vi "数据发送组合-20200825 (子VI).vi"(10 "枚举":T2(ring), 11 "插值后的数组元素":T1) -> (3 "字符串":string)   [LabVIEW 2016, in "数据传输系统-06.lvlib"]
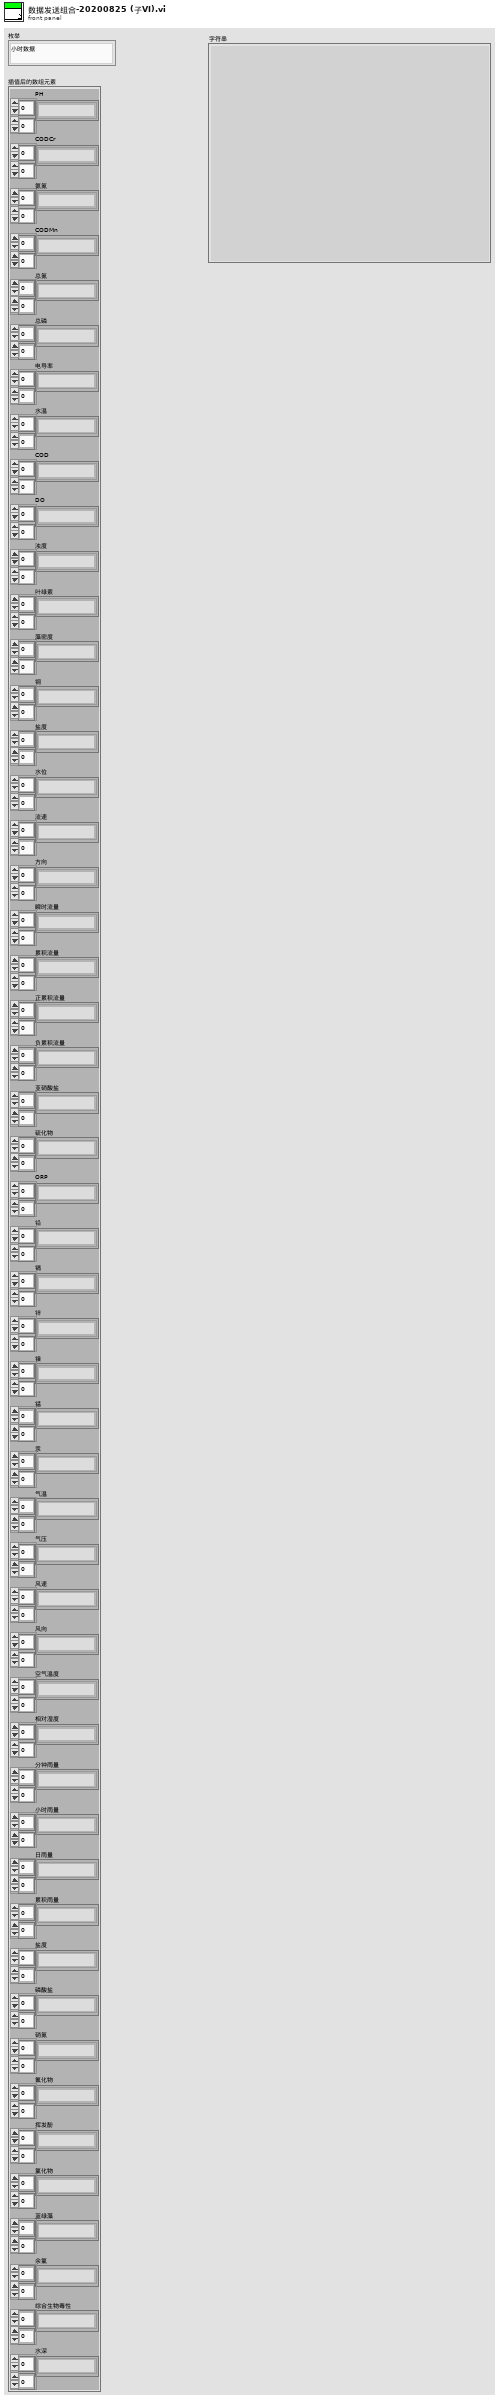
[diagram p1: front panel]
types:
  T1 = cluster{"PH":string[][], "CODCr":string[][], "氨氮":string[][], "CODMn":string[][], "总氮":string[][], "总磷":string[][], "电导率":string[][], "水温":string[][], "COD":string[][], "DO":string[][], "浊度":string[][], "叶绿素":string[][], "藻密度":string[][], "铜":string[][], "盐度":string[][], "水位":string[][], "流速":string[][], "方向":string[][], "瞬时流量":string[][], "累积流量":string[][], "正累积流量":string[][], "负累积流量":string[][], "亚硝酸盐":string[][], "硫化物":string[][], "ORP":string[][], "铅":string[][], "镉":string[][], "锌":string[][], "镍":string[][], "锰":string[][], "汞":string[][], "气温":string[][], "气压":string[][], "风速":string[][], "风向":string[][], "空气温度":string[][], "相对湿度":string[][], "分钟雨量":string[][], "小时雨量":string[][], "日雨量":string[][], "累积雨量":string[][], "盐度":string[][], "磷酸盐":string[][], "硝氮":string[][], "氟化物":string[][], "挥发酚":string[][], "氯化物":string[][], "蓝绿藻":string[][], "余氯":string[][], "综合生物毒性":string[][], "水深":string[][]}
  T2 = enum16{"小时数据", "实时数据", "平行样测试", "集成干预测试", "加标回收测试", "核查数据", "空白零点跨度数据", "提取小时数据", "提取实时数据", "操作日志", "仪器参数", "3090仪器参数", "提取仪器参数", "报警信息"}
  T3 = cluster{"CODMn":dbl, "CODCr":dbl, "DO":dbl, "铜":dbl, "PH":dbl, "氨氮":dbl, "比电导率":dbl, "水温":dbl, "COD":dbl, "浊度":dbl, "总氮":dbl, "总磷":dbl, "叶绿素a":dbl, "藻密度":dbl, "水位":dbl, "流速":dbl, "方向":dbl, "瞬时流量":dbl, "累积流量":dbl, "正累积流量":dbl, "负累积流量":dbl, "亚硝酸盐":dbl, "硫化物":dbl, "ORP":dbl, "铅":dbl, "镉":dbl, "锌":dbl, "镍":dbl, "锰":dbl, "汞":dbl, "气温":dbl, "气压":dbl, "风速":dbl, "风向":dbl, "空气温度":dbl, "相对湿度":dbl, "分钟雨量":dbl, "小时雨量":dbl, "日雨量":dbl, "累积雨量":dbl, "盐度":dbl, "磷酸盐":dbl, "硝氮":dbl, "氟化物":dbl, "挥发酚":dbl, "氯化物":dbl, "蓝绿藻":dbl, "余氯":dbl, "综合生物毒性":dbl, "艏向":dbl, "横摇":dbl, "纵摇":dbl, "分层标志":dbl, "层状态1":dbl, "层状态2":dbl, "水平平均流速":dbl, "流向":dbl, "北向流速分量":dbl, "东向流速分量":dbl, "垂直流速分量":dbl, "最大波高":dbl, "最大波周期":dbl, "1/10波高":dbl, "1/10波周期":dbl, "有效波高":dbl, "有效波周期":dbl, "平均波高":dbl, "平均波周期":dbl, "波向":dbl, "波个数":dbl, "水深":dbl, "X轴流速":dbl, "Y轴流速":dbl, "信号强度":dbl, "电压":dbl, "悬浮物":dbl}
  T4 = cluster{"CODMn":string, "CODCr":string, "DO":string, "铜":string, "PH":string, "氨氮":string, "比电导率":string, "水温":string, "COD":string, "浊度":string, "总氮":string, "总磷":string, "叶绿素a":string, "藻密度":string, "水位":string, "流速":string, "方向":string, "瞬时流量":string, "累积流量":string, "正累积流量":string, "负累积流量":string, "亚硝酸盐":string, "硫化物":string, "ORP":string, "铅":string, "镉":string, "锌":string, "镍":string, "锰":string, "汞":string, "气温":string, "气压":string, "风速":string, "风向":string, "空气温度":string, "相对湿度":string, "分钟雨量":string, "小时雨量":string, "日雨量":string, "累积雨量":string, "盐度":string, "磷酸盐":string, "硝氮":string, "氟化物":string, "挥发酚":string, "氯化物":string, "蓝绿藻":string, "余氯":string, "综合生物毒性":string, "艏向":string, "横摇":string, "纵摇":string, "分层标志":string, "层状态1":string, "层状态2":string, "水平平均流速":string, "流向":string, "北向流速分量":string, "东向流速分量":string, "垂直流速分量":string, "最大波高":string, "最大波周期":string, "1/10波高":string, "1/10波周期":string, "有效波高":string, "有效波周期":string, "平均波高":string, "平均波周期":string, "波向":string, "波个数":string, "水深":string, "X轴流速":string, "Y轴流速":string, "信号强度":string, "电压":string, "悬浮物":string}
  T5 = typedef "数据传输系统-06.lvlib/应用环境.ctl" = enum16{"STD", "GB212", "婉仪平台"}
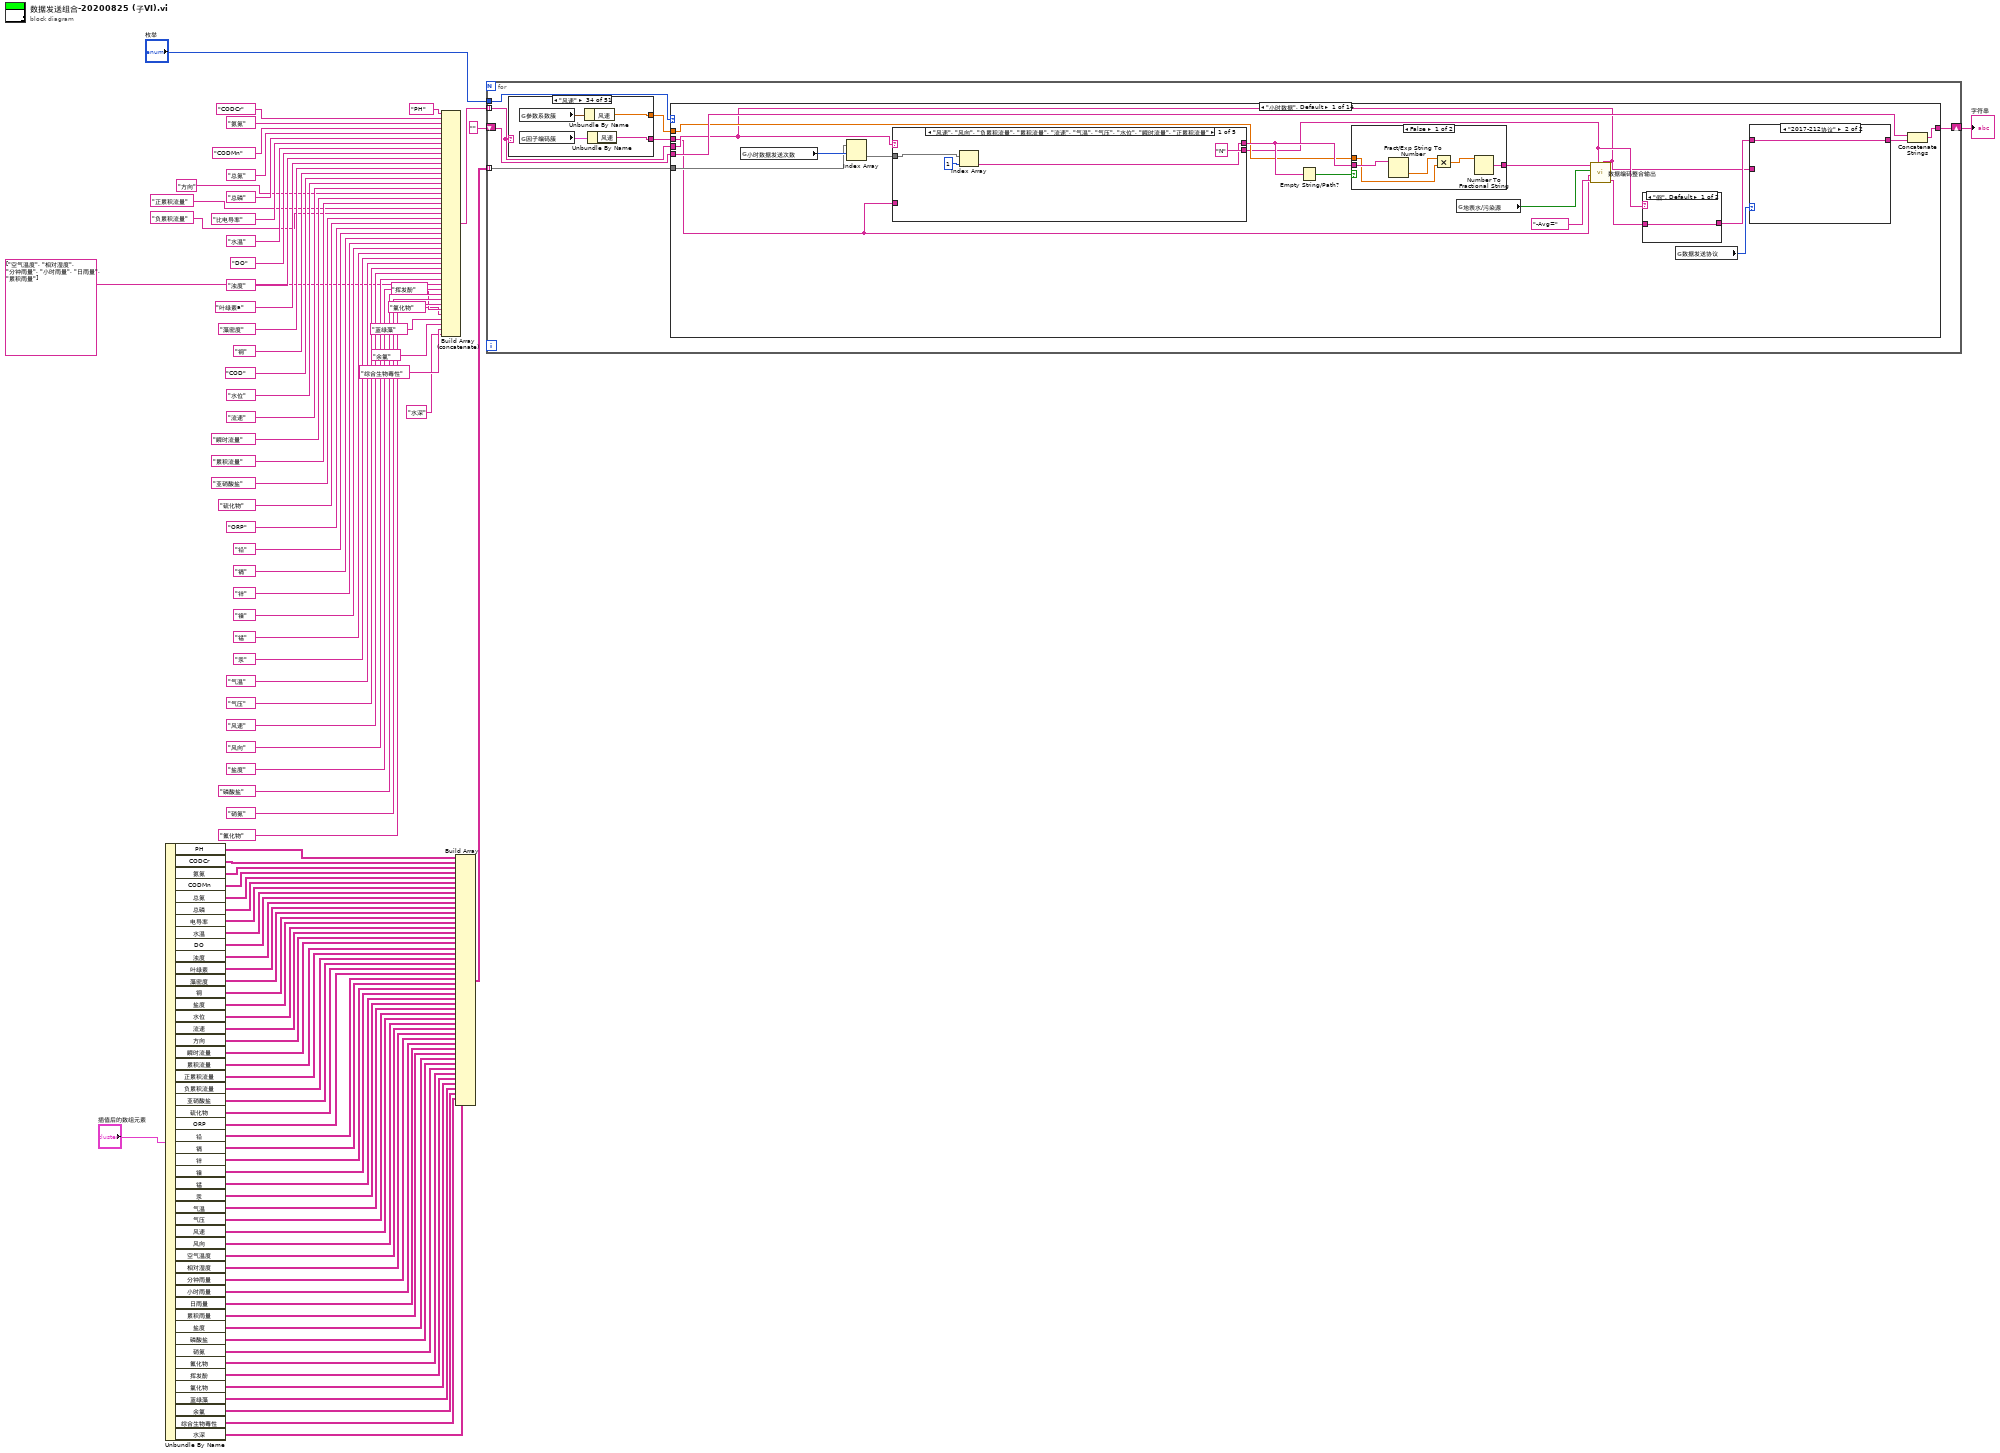
[diagram p0: block diagram]
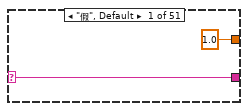
[diagram p2: hidden frame]
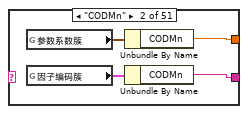
[diagram p3: hidden frame]
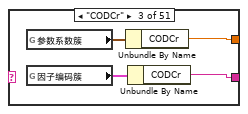
[diagram p4: hidden frame]
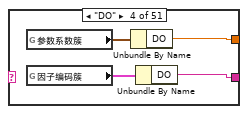
[diagram p5: hidden frame]
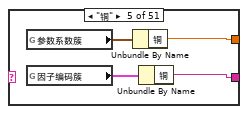
[diagram p6: hidden frame]
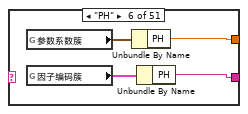
[diagram p7: hidden frame]
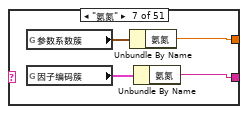
[diagram p8: hidden frame]
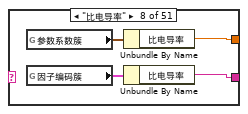
[diagram p9: hidden frame]
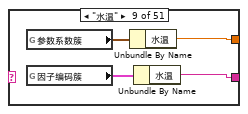
[diagram p10: hidden frame]
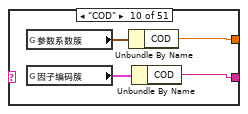
[diagram p11: hidden frame]
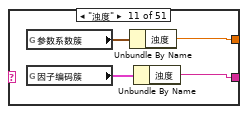
[diagram p12: hidden frame]
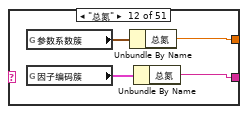
[diagram p13: hidden frame]
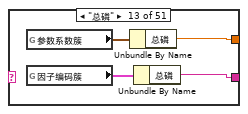
[diagram p14: hidden frame]
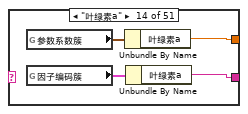
[diagram p15: hidden frame]
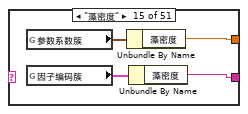
[diagram p16: hidden frame]
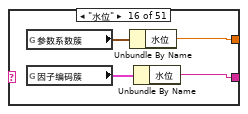
[diagram p17: hidden frame]
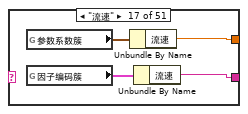
[diagram p18: hidden frame]
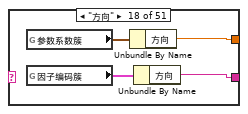
[diagram p19: hidden frame]
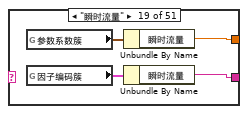
[diagram p20: hidden frame]
diagram:
  n1 = Unbundle By Name("插值后的数组元素") -> ("PH"=w101:string[][], "CODCr"=w100:string[][], "氨氮"=w99:string[][], "CODMn"=w98:string[][], "总氮"=w97:string[][], "总磷"=w96:string[][], "电导率"=w95:string[][], "水温"=w94:string[][], "DO"=w93:string[][], "浊度"=w92:string[][], "叶绿素"=w91:string[][], "藻密度"=w90:string[][], "铜"=w89:string[][], "盐度"=w88:string[][], "水位"=w87:string[][], "流速"=w86:string[][], "方向"=w11:string[][], "瞬时流量"=w10:string[][], "累积流量"=w12:string[][], "正累积流量"=w9:string[][], "负累积流量"=w8:string[][], "亚硝酸盐"=w85:string[][], "硫化物"=w84:string[][], "ORP"=w83:string[][], "铅"=w82:string[][], "镉"=w81:string[][], "锌"=w80:string[][], "镍"=w79:string[][], "锰"=w78:string[][], "汞"=w77:string[][], "气温"=w41:string[][], "气压"=w42:string[][], "风速"=w43:string[][], "风向"=w44:string[][], "空气温度"=w36:string[][], "相对湿度"=w19:string[][], "分钟雨量"=w18:string[][], "小时雨量"=w17:string[][], "日雨量"=w16:string[][], "累积雨量"=w15:string[][], "盐度"=w20:string[][], "磷酸盐"=w21:string[][], "硝氮"=w35:string[][], "氟化物"=w31:string[][], "挥发酚"=w29:string[][], "氯化物"=w28:string[][], "蓝绿藻"=w24:string[][], "余氯"=w22:string[][], "综合生物毒性"=w7:string[][], "水深"=w1:string[][])
  n2 = Build Array (concatenate)("PH" ("污染物编码"), "CODCr" ("污染物编码"), "氨氮" ("污染物编码"), "CODMn" ("污染物编码"), "总氮" ("污染物编码"), "总磷" ("污染物编码"), "比电导率" ("污染物编码"), "水温" ("污染物编码"), "DO" ("污染物编码"), "浊度" ("污染物编码"), "叶绿素a" ("污染物编码"), "藻密度" ("污染物编码"), "铜" ("污染物编码"), "COD" ("污染物编码"), "水位" ("污染物编码"), "流速" ("污染物编码"), "方向", "瞬时流量" ("污染物编码"), "累积流量" ("污染物编码"), "正累积流量", "负累积流量", "亚硝酸盐" ("污染物编码"), "硫化物" ("污染物编码"), "ORP" ("污染物编码"), "铅" ("污染物编码"), "镉" ("污染物编码"), "锌" ("污染物编码"), "镍" ("污染物编码"), "锰" ("污染物编码"), "汞" ("污染物编码"), "气温" ("污染物编码"), "气压" ("污染物编码"), "风速" ("污染物编码"), "风向" ("污染物编码"), string[] ["空气温度", "相对湿度", "分钟雨量", "小时雨量", "日雨量", "累积雨量"], "盐度" ("污染物编码"), "磷酸盐" ("污染物编码"), "硝氮" ("污染物编码"), "氟化物" ("污染物编码"), "挥发酚" ("污染物编码"), "氯化物" ("污染物编码"), "蓝绿藻" ("污染物编码"), "余氯" ("污染物编码"), "综合生物毒性", "水深") -> (w48:string[])
  n3 = Build Array(w101, w100, w99, w98, w97, w96, w95, w94, w93, w92, w91, w90, w89, w88, w87, w86, w11, w10, w12, w9, w8, w85, w84, w83, w82, w81, w80, w79, w78, w77, w41, w42, w43, w44, w36, w19, w18, w17, w16, w15, w20, w21, w35, w31, w29, w28, w24, w22, w7, w1) -> (w76:string[][][])
  n4 = for {
    tunnel: w76 -> [w108] mode=indexing
    tunnel: w48 -> [w103] mode=indexing
    shift-right: [w107] -> w46
    shift-left: "" -> [w102]
    tunnel: "枚举" -> [w106]
    n5 = case shown="\"风速\"" w103 {
      selector: w103 -> [w110 _ _ _ _ _ _ _ _ _ _ _ _ _ _ _ _ _ _ _ _ _ _ _ _ _ _ _ _ _ _ _ _ _ _ _ _ _ _ _ _ _ _ _ _ _ _ _ _ _ _]
      tunnel: [w110 w113 w117 w121 w125 w129 w133 w137 w141 w145 w149 w153 w157 w161 w165 w169 w173 w177 w181 w185 w189 w193 w197 w201 w205 w209 w213 w217 w221 w225 w229 w233 w237 w241 w245 w249 w253 w257 w261 w265 w269 w273 w277 w281 w285 w289 w293 w297 w301 w305 w309] -> w105
      tunnel: [1.0 ("风向") w111 w115 w119 w123 w127 w131 w135 w139 w143 w147 w151 w155 w159 w163 w167 w171 w175 w179 w183 w187 w191 w195 w199 w203 w207 w211 w215 w219 w223 w227 w231 w235 w239 w243 w247 w251 w255 w259 w263 w267 w271 w275 w279 w283 w287 w291 w295 w299 w303 w307] -> w104
      frame "假", Default {
      }
      frame "CODMn" {
        n6 = global read "断电保存全局.vi" "参数系数簇"() -> (w112:T3)
        n7 = global read "断电保存全局.vi" "因子编码簇"() -> (w114:T4)
        n8 = Unbundle By Name(w112) -> ("CODMn"=w111:dbl)
        n9 = Unbundle By Name(w114) -> ("CODMn"=w113:string)
      }
      frame "CODCr" {
        n10 = global read "断电保存全局.vi" "参数系数簇"() -> (w116:T3)
        n11 = global read "断电保存全局.vi" "因子编码簇"() -> (w118:T4)
        n12 = Unbundle By Name(w116) -> ("CODCr"=w115:dbl)
        n13 = Unbundle By Name(w118) -> ("CODCr"=w117:string)
      }
      frame "DO" {
        n14 = global read "断电保存全局.vi" "参数系数簇"() -> (w120:T3)
        n15 = global read "断电保存全局.vi" "因子编码簇"() -> (w122:T4)
        n16 = Unbundle By Name(w120) -> ("DO"=w119:dbl)
        n17 = Unbundle By Name(w122) -> ("DO"=w121:string)
      }
      frame "铜" {
        n18 = global read "断电保存全局.vi" "参数系数簇"() -> (w124:T3)
        n19 = global read "断电保存全局.vi" "因子编码簇"() -> (w126:T4)
        n20 = Unbundle By Name(w124) -> ("铜"=w123:dbl)
        n21 = Unbundle By Name(w126) -> ("铜"=w125:string)
      }
      frame "PH" {
        n22 = global read "断电保存全局.vi" "参数系数簇"() -> (w128:T3)
        n23 = global read "断电保存全局.vi" "因子编码簇"() -> (w130:T4)
        n24 = Unbundle By Name(w128) -> ("PH"=w127:dbl)
        n25 = Unbundle By Name(w130) -> ("PH"=w129:string)
      }
      frame "氨氮" {
        n26 = global read "断电保存全局.vi" "参数系数簇"() -> (w132:T3)
        n27 = global read "断电保存全局.vi" "因子编码簇"() -> (w134:T4)
        n28 = Unbundle By Name(w132) -> ("氨氮"=w131:dbl)
        n29 = Unbundle By Name(w134) -> ("氨氮"=w133:string)
      }
      frame "比电导率" {
        n30 = global read "断电保存全局.vi" "参数系数簇"() -> (w136:T3)
        n31 = global read "断电保存全局.vi" "因子编码簇"() -> (w138:T4)
        n32 = Unbundle By Name(w136) -> ("比电导率"=w135:dbl)
        n33 = Unbundle By Name(w138) -> ("比电导率"=w137:string)
      }
      frame "水温" {
        n34 = global read "断电保存全局.vi" "参数系数簇"() -> (w140:T3)
        n35 = global read "断电保存全局.vi" "因子编码簇"() -> (w142:T4)
        n36 = Unbundle By Name(w140) -> ("水温"=w139:dbl)
        n37 = Unbundle By Name(w142) -> ("水温"=w141:string)
      }
      frame "COD" {
        n38 = global read "断电保存全局.vi" "参数系数簇"() -> (w144:T3)
        n39 = global read "断电保存全局.vi" "因子编码簇"() -> (w146:T4)
        n40 = Unbundle By Name(w144) -> ("COD"=w143:dbl)
        n41 = Unbundle By Name(w146) -> ("COD"=w145:string)
      }
      frame "浊度" {
        n42 = global read "断电保存全局.vi" "参数系数簇"() -> (w148:T3)
        n43 = global read "断电保存全局.vi" "因子编码簇"() -> (w150:T4)
        n44 = Unbundle By Name(w148) -> ("浊度"=w147:dbl)
        n45 = Unbundle By Name(w150) -> ("浊度"=w149:string)
      }
      frame "总氮" {
        n46 = global read "断电保存全局.vi" "参数系数簇"() -> (w152:T3)
        n47 = global read "断电保存全局.vi" "因子编码簇"() -> (w154:T4)
        n48 = Unbundle By Name(w152) -> ("总氮"=w151:dbl)
        n49 = Unbundle By Name(w154) -> ("总氮"=w153:string)
      }
      frame "总磷" {
        n50 = global read "断电保存全局.vi" "参数系数簇"() -> (w156:T3)
        n51 = global read "断电保存全局.vi" "因子编码簇"() -> (w158:T4)
        n52 = Unbundle By Name(w156) -> ("总磷"=w155:dbl)
        n53 = Unbundle By Name(w158) -> ("总磷"=w157:string)
      }
      frame "叶绿素a" {
        n54 = global read "断电保存全局.vi" "参数系数簇"() -> (w160:T3)
        n55 = global read "断电保存全局.vi" "因子编码簇"() -> (w162:T4)
        n56 = Unbundle By Name(w160) -> ("叶绿素a"=w159:dbl)
        n57 = Unbundle By Name(w162) -> ("叶绿素a"=w161:string)
      }
      frame "藻密度" {
        n58 = global read "断电保存全局.vi" "参数系数簇"() -> (w164:T3)
        n59 = global read "断电保存全局.vi" "因子编码簇"() -> (w166:T4)
        n60 = Unbundle By Name(w164) -> ("藻密度"=w163:dbl)
        n61 = Unbundle By Name(w166) -> ("藻密度"=w165:string)
      }
      frame "水位" {
        n62 = global read "断电保存全局.vi" "参数系数簇"() -> (w168:T3)
        n63 = global read "断电保存全局.vi" "因子编码簇"() -> (w170:T4)
        n64 = Unbundle By Name(w168) -> ("水位"=w167:dbl)
        n65 = Unbundle By Name(w170) -> ("水位"=w169:string)
      }
      frame "流速" {
        n66 = global read "断电保存全局.vi" "参数系数簇"() -> (w172:T3)
        n67 = global read "断电保存全局.vi" "因子编码簇"() -> (w174:T4)
        n68 = Unbundle By Name(w172) -> ("流速"=w171:dbl)
        n69 = Unbundle By Name(w174) -> ("流速"=w173:string)
      }
      frame "方向" {
        n70 = global read "断电保存全局.vi" "参数系数簇"() -> (w176:T3)
        n71 = global read "断电保存全局.vi" "因子编码簇"() -> (w178:T4)
        n72 = Unbundle By Name(w176) -> ("方向"=w175:dbl)
        n73 = Unbundle By Name(w178) -> ("方向"=w177:string)
      }
      frame "瞬时流量" {
        n74 = global read "断电保存全局.vi" "参数系数簇"() -> (w180:T3)
        n75 = global read "断电保存全局.vi" "因子编码簇"() -> (w182:T4)
        n76 = Unbundle By Name(w180) -> ("瞬时流量"=w179:dbl)
        n77 = Unbundle By Name(w182) -> ("瞬时流量"=w181:string)
      }
      frame "累积流量" {
        n78 = global read "断电保存全局.vi" "参数系数簇"() -> (w184:T3)
        n79 = global read "断电保存全局.vi" "因子编码簇"() -> (w186:T4)
        n80 = Unbundle By Name(w184) -> ("累积流量"=w183:dbl)
        n81 = Unbundle By Name(w186) -> ("累积流量"=w185:string)
      }
      frame "正累积流量" {
        n82 = global read "断电保存全局.vi" "参数系数簇"() -> (w188:T3)
        n83 = global read "断电保存全局.vi" "因子编码簇"() -> (w190:T4)
        n84 = Unbundle By Name(w188) -> ("正累积流量"=w187:dbl)
        n85 = Unbundle By Name(w190) -> ("正累积流量"=w189:string)
      }
      frame "负累积流量" {
        n86 = global read "断电保存全局.vi" "参数系数簇"() -> (w192:T3)
        n87 = global read "断电保存全局.vi" "因子编码簇"() -> (w194:T4)
        n88 = Unbundle By Name(w192) -> ("负累积流量"=w191:dbl)
        n89 = Unbundle By Name(w194) -> ("负累积流量"=w193:string)
      }
      frame "亚硝酸盐" {
        n90 = global read "断电保存全局.vi" "参数系数簇"() -> (w196:T3)
        n91 = global read "断电保存全局.vi" "因子编码簇"() -> (w198:T4)
        n92 = Unbundle By Name(w196) -> ("亚硝酸盐"=w195:dbl)
        n93 = Unbundle By Name(w198) -> ("亚硝酸盐"=w197:string)
      }
      frame "硫化物" {
        n94 = global read "断电保存全局.vi" "参数系数簇"() -> (w200:T3)
        n95 = global read "断电保存全局.vi" "因子编码簇"() -> (w202:T4)
        n96 = Unbundle By Name(w200) -> ("硫化物"=w199:dbl)
        n97 = Unbundle By Name(w202) -> ("硫化物"=w201:string)
      }
      frame "ORP" {
        n98 = global read "断电保存全局.vi" "参数系数簇"() -> (w204:T3)
        n99 = global read "断电保存全局.vi" "因子编码簇"() -> (w206:T4)
        n100 = Unbundle By Name(w204) -> ("ORP"=w203:dbl)
        n101 = Unbundle By Name(w206) -> ("ORP"=w205:string)
      }
      frame "铅" {
        n102 = global read "断电保存全局.vi" "参数系数簇"() -> (w208:T3)
        n103 = global read "断电保存全局.vi" "因子编码簇"() -> (w210:T4)
        n104 = Unbundle By Name(w208) -> ("铅"=w207:dbl)
        n105 = Unbundle By Name(w210) -> ("铅"=w209:string)
      }
      frame "镉" {
        n106 = global read "断电保存全局.vi" "参数系数簇"() -> (w212:T3)
        n107 = global read "断电保存全局.vi" "因子编码簇"() -> (w214:T4)
        n108 = Unbundle By Name(w212) -> ("镉"=w211:dbl)
        n109 = Unbundle By Name(w214) -> ("镉"=w213:string)
      }
      frame "锌" {
        n110 = global read "断电保存全局.vi" "参数系数簇"() -> (w216:T3)
        n111 = global read "断电保存全局.vi" "因子编码簇"() -> (w218:T4)
        n112 = Unbundle By Name(w216) -> ("锌"=w215:dbl)
        n113 = Unbundle By Name(w218) -> ("锌"=w217:string)
      }
      frame "镍" {
        n114 = global read "断电保存全局.vi" "参数系数簇"() -> (w220:T3)
        n115 = global read "断电保存全局.vi" "因子编码簇"() -> (w222:T4)
        n116 = Unbundle By Name(w220) -> ("镍"=w219:dbl)
        n117 = Unbundle By Name(w222) -> ("镍"=w221:string)
      }
      frame "锰" {
        n118 = global read "断电保存全局.vi" "参数系数簇"() -> (w224:T3)
        n119 = global read "断电保存全局.vi" "因子编码簇"() -> (w226:T4)
        n120 = Unbundle By Name(w224) -> ("锰"=w223:dbl)
        n121 = Unbundle By Name(w226) -> ("锰"=w225:string)
      }
      frame "汞" {
        n122 = global read "断电保存全局.vi" "参数系数簇"() -> (w228:T3)
        n123 = global read "断电保存全局.vi" "因子编码簇"() -> (w230:T4)
        n124 = Unbundle By Name(w228) -> ("汞"=w227:dbl)
        n125 = Unbundle By Name(w230) -> ("汞"=w229:string)
      }
      frame "气温" {
        n126 = global read "断电保存全局.vi" "参数系数簇"() -> (w232:T3)
        n127 = global read "断电保存全局.vi" "因子编码簇"() -> (w234:T4)
        n128 = Unbundle By Name(w232) -> ("气温"=w231:dbl)
        n129 = Unbundle By Name(w234) -> ("气温"=w233:string)
      }
      frame "气压" {
        n130 = global read "断电保存全局.vi" "参数系数簇"() -> (w236:T3)
        n131 = global read "断电保存全局.vi" "因子编码簇"() -> (w238:T4)
        n132 = Unbundle By Name(w236) -> ("气压"=w235:dbl)
        n133 = Unbundle By Name(w238) -> ("气压"=w237:string)
      }
      frame "风速" {
        n134 = global read "断电保存全局.vi" "参数系数簇"() -> (w240:T3)
        n135 = global read "断电保存全局.vi" "因子编码簇"() -> (w242:T4)
        n136 = Unbundle By Name(w240) -> ("风速"=w239:dbl)
        n137 = Unbundle By Name(w242) -> ("风速"=w241:string)
      }
      frame "风向" {
        n138 = global read "断电保存全局.vi" "参数系数簇"() -> (w244:T3)
        n139 = global read "断电保存全局.vi" "因子编码簇"() -> (w246:T4)
        n140 = Unbundle By Name(w244) -> ("风向"=w243:dbl)
        n141 = Unbundle By Name(w246) -> ("风向"=w245:string)
      }
      frame "空气温度" {
        n142 = global read "断电保存全局.vi" "参数系数簇"() -> (w248:T3)
        n143 = global read "断电保存全局.vi" "因子编码簇"() -> (w250:T4)
        n144 = Unbundle By Name(w248) -> ("空气温度"=w247:dbl)
        n145 = Unbundle By Name(w250) -> ("空气温度"=w249:string)
      }
      frame "相对湿度" {
        n146 = global read "断电保存全局.vi" "参数系数簇"() -> (w252:T3)
        n147 = global read "断电保存全局.vi" "因子编码簇"() -> (w254:T4)
        n148 = Unbundle By Name(w252) -> ("相对湿度"=w251:dbl)
        n149 = Unbundle By Name(w254) -> ("相对湿度"=w253:string)
      }
      frame "分钟雨量" {
        n150 = global read "断电保存全局.vi" "参数系数簇"() -> (w256:T3)
        n151 = global read "断电保存全局.vi" "因子编码簇"() -> (w258:T4)
        n152 = Unbundle By Name(w256) -> ("分钟雨量"=w255:dbl)
        n153 = Unbundle By Name(w258) -> ("分钟雨量"=w257:string)
      }
      frame "小时雨量" {
        n154 = global read "断电保存全局.vi" "参数系数簇"() -> (w260:T3)
        n155 = global read "断电保存全局.vi" "因子编码簇"() -> (w262:T4)
        n156 = Unbundle By Name(w260) -> ("小时雨量"=w259:dbl)
        n157 = Unbundle By Name(w262) -> ("小时雨量"=w261:string)
      }
      frame "日雨量" {
        n158 = global read "断电保存全局.vi" "参数系数簇"() -> (w264:T3)
        n159 = global read "断电保存全局.vi" "因子编码簇"() -> (w266:T4)
        n160 = Unbundle By Name(w264) -> ("日雨量"=w263:dbl)
        n161 = Unbundle By Name(w266) -> ("日雨量"=w265:string)
      }
      frame "累积雨量" {
        n162 = global read "断电保存全局.vi" "参数系数簇"() -> (w268:T3)
        n163 = global read "断电保存全局.vi" "因子编码簇"() -> (w270:T4)
        n164 = Unbundle By Name(w268) -> ("累积雨量"=w267:dbl)
        n165 = Unbundle By Name(w270) -> ("累积雨量"=w269:string)
      }
      frame "盐度" {
        n166 = global read "断电保存全局.vi" "参数系数簇"() -> (w272:T3)
        n167 = global read "断电保存全局.vi" "因子编码簇"() -> (w274:T4)
        n168 = Unbundle By Name(w272) -> ("盐度"=w271:dbl)
        n169 = Unbundle By Name(w274) -> ("盐度"=w273:string)
      }
      frame "磷酸盐" {
        n170 = global read "断电保存全局.vi" "参数系数簇"() -> (w276:T3)
        n171 = global read "断电保存全局.vi" "因子编码簇"() -> (w278:T4)
        n172 = Unbundle By Name(w276) -> ("磷酸盐"=w275:dbl)
        n173 = Unbundle By Name(w278) -> ("磷酸盐"=w277:string)
      }
      frame "硝氮" {
        n174 = global read "断电保存全局.vi" "参数系数簇"() -> (w280:T3)
        n175 = global read "断电保存全局.vi" "因子编码簇"() -> (w282:T4)
        n176 = Unbundle By Name(w280) -> ("硝氮"=w279:dbl)
        n177 = Unbundle By Name(w282) -> ("硝氮"=w281:string)
      }
      frame "氟化物" {
        n178 = global read "断电保存全局.vi" "参数系数簇"() -> (w284:T3)
        n179 = global read "断电保存全局.vi" "因子编码簇"() -> (w286:T4)
        n180 = Unbundle By Name(w284) -> ("氟化物"=w283:dbl)
        n181 = Unbundle By Name(w286) -> ("氟化物"=w285:string)
      }
      frame "挥发酚" {
        n182 = global read "断电保存全局.vi" "参数系数簇"() -> (w288:T3)
        n183 = global read "断电保存全局.vi" "因子编码簇"() -> (w290:T4)
        n184 = Unbundle By Name(w288) -> ("挥发酚"=w287:dbl)
        n185 = Unbundle By Name(w290) -> ("挥发酚"=w289:string)
      }
      frame "氯化物" {
        n186 = global read "断电保存全局.vi" "参数系数簇"() -> (w292:T3)
        n187 = global read "断电保存全局.vi" "因子编码簇"() -> (w294:T4)
        n188 = Unbundle By Name(w292) -> ("氯化物"=w291:dbl)
        n189 = Unbundle By Name(w294) -> ("氯化物"=w293:string)
      }
      frame "蓝绿藻" {
        n190 = global read "断电保存全局.vi" "参数系数簇"() -> (w296:T3)
        n191 = global read "断电保存全局.vi" "因子编码簇"() -> (w298:T4)
        n192 = Unbundle By Name(w296) -> ("蓝绿藻"=w295:dbl)
        n193 = Unbundle By Name(w298) -> ("蓝绿藻"=w297:string)
      }
      frame "余氯" {
        n194 = global read "断电保存全局.vi" "参数系数簇"() -> (w300:T3)
        n195 = global read "断电保存全局.vi" "因子编码簇"() -> (w302:T4)
        n196 = Unbundle By Name(w300) -> ("余氯"=w299:dbl)
        n197 = Unbundle By Name(w302) -> ("余氯"=w301:string)
      }
      frame "综合生物毒性" {
        n198 = global read "断电保存全局.vi" "参数系数簇"() -> (w304:T3)
        n199 = global read "断电保存全局.vi" "因子编码簇"() -> (w306:T4)
        n200 = Unbundle By Name(w304) -> ("综合生物毒性"=w303:dbl)
        n201 = Unbundle By Name(w306) -> ("综合生物毒性"=w305:string)
      }
      frame "水深" {
        n202 = global read "断电保存全局.vi" "参数系数簇"() -> (w308:T3)
        n203 = global read "断电保存全局.vi" "因子编码簇"() -> (w310:T4)
        n204 = Unbundle By Name(w308) -> ("水深"=w307:dbl)
        n205 = Unbundle By Name(w310) -> ("水深"=w309:string)
      }
    }
    n206 = case shown="\"小时数据\", Default" w106 {
      tunnel: w108 -> [w326 w386 w423 w432 w487 w493 w505 w530 w553 w590 w608 w615 w625 w647]
      tunnel: w105 -> [w312 w373 w422 w433 w483 w492 w504 w524 w552 w578 w606 w613 w624 w650]
      tunnel: [w325 w383 w424 w430 w488 w489 w501 w521 w551 w585 w603 w612 w620 w636] -> w107
      tunnel: w102 -> [w324 w384 w426 w431 w484 w491 w502 w522 w554 w586 w604 w614 w621 w631]
      tunnel: w103 -> [w313 w374 _ w427 _ _ _ w515 w545 _ _ _ _ w645]
      tunnel: w104 -> [w319 w376 _ w428 _ _ _ w517 w547 _ _ _ _ _]
      frame "小时数据", Default {
        n207 = global read "全局 小时数据发送次数.vi" "小时数据发送次数"() -> (w328:i32)
        n208 = Index Array(array=w326, index (row)=w328) -> (element=w311:string[])  [unwired: 1 in]
        n209 = case shown="\"风速\", \"风向\", \"负累积流量\", \"累积流量\", \"流速\", \"气温\", \"气压\", \"水位\", \"瞬时流量\", \"正累积流量\"" w313 {
          tunnel: w311 -> [w340 w344 w349 w355 w358]
          tunnel: [w337 w341 "" w352 w356] -> w320
          tunnel: ["N" ("字符串") "N" ("字符串") "N" ("字符串") "N" ("字符串") w357] -> w316
          tunnel: w312 -> [_ _ _ _ _]
          frame "风速", "风向", "负累积流量", "累积流量", "流速", "气温", "气压", "水位", "瞬时流量", "正累积流量" {
            n210 = Index Array(array=w340, index=1 ("索引")) -> (element=w337:string)
          }
          frame "水深" {
            n211 = Index Array(array=w344, index=1 ("索引")) -> (element=w341:string)
          }
          frame "方向" {
            n212 = Index Array(array=w349, index=1 ("索引")) -> (element=w346:string)
            n213 = case shown="\"负向\"" w346 {
              tunnel: ["1" "0"] -> _
              frame "负向" {
              }
              frame "正向", Default {
              }
            }
          }
          frame "分钟雨量", "空气温度", "累积雨量", "日雨量", "相对湿度", "小时雨量" {
            n214 = Index Array(array=w355, index=1 ("索引")) -> (element=w352:string)
          }
          frame "", Default {
            n215 = Index Array(array=w358, index #1=2 ("索引"), index #2=3 ("索引"), index #3=5 ("索引")) -> (element #1=w361:string, element #2=w360:string, element #3=w357:string)
            n216 = case shown="\"M\"" w361 {
              tunnel: [w364 ""] -> w356
              tunnel: w360 -> [w364 _]
              frame "N", Default {
              }
              frame "M" {
              }
            }
          }
        }
        n217 = Empty String/Path?(string/path=w320) -> (empty?=w321:bool)
        n218 = case shown="False" w321 {
          tunnel: w320 -> [w334 w336]
          tunnel: w319 -> [w333 _]
          tunnel: [w331 w336] -> w318
          frame False {
            n219 = Fract/Exp String To Number(string=w334) -> (number=w335:dbl)  [unwired: 3 in, 1 out]
            n220 = Multiply(x=w335, y=w333) -> (x*y=w332:dbl)
            n221 = Number To Fractional String(number=w332) -> (F-format string=w331:string)  [unwired: 3 in]
          }
          frame True {
            # "空"
          }
        }
        n222 = global read "断电保存全局.vi" "地表水/污染源"() -> (w317:bool)
        n223 = call "数据编码整合输出.vi"("table"=w313, "数据标识"=w316, "数据类型"="-Avg=", "污染物编码"=w312, "地表水/污染源"=w317, "数据值"=w318) -> ("编码输出"=w315:string)  [unwired: 5 in]
        n224 = case shown="\"假\", Default" w316 {
          tunnel: w315 -> [w329 _]
          tunnel: [w329 ""] -> w314
          frame "假", Default {
          }
          frame "pf" {
            # "pf不传小时数据"
          }
        }
        n225 = global read "断电保存全局.vi" "数据发送协议"() -> (w323:enum16{"2005-212协议", "2017-212协议"})
        n226 = case shown="\"2017-212协议\"" w323 {
          tunnel: w313 -> [w368 _]
          tunnel: w314 -> [w366 w372]
          tunnel: [w367 w372] -> w322
          frame "2005-212协议", Default {
            n227 = case shown="\"假\", Default" w368 {
              tunnel: [w369 "" ""] -> w367
              tunnel: w366 -> [w369 _ _]
              frame "假", Default {
              }
              frame "风速", "风向", "负累积流量", "累积流量", "流速", "气温", "气压", "水位", "瞬时流量", "正累积流量" {
              }
              frame "分钟雨量", "空气温度", "累积雨量", "日雨量", "相对湿度", "小时雨量" {
              }
            }
          }
          frame "2017-212协议" {
          }
        }
        n228 = Concatenate Strings(w324, w322) -> (w325:string)
      }
      frame "实时数据" {
        n229 = global read "全局 小时数据发送次数.vi" "小时数据发送次数"() -> (w387:i32)
        n230 = Index Array(array=w386, index (row)=w387) -> (element=w388:string[])  [unwired: 1 in]
        n231 = case shown="\"\", Default" w374 {
          tunnel: w388 -> [w397 w403 w405 w411]
          tunnel: [w396 w401 w404 w410] -> w378
          tunnel: ["N" ("字符串") "N" ("字符串") "N" ("字符串") w408] -> w385
          frame "方向", "负累积流量", "累积流量", "流速", "水位", "瞬时流量", "正累积流量" {
            n232 = Index Array(array=w397, index=1 ("索引")) -> (element=w396:string)
          }
          frame "分钟雨量", "空气温度", "累积雨量", "日雨量", "相对湿度", "小时雨量" {
            n233 = Index Array(array=w403, index=1 ("索引")) -> (element=w401:string)
          }
          frame "风速", "风向", "气温", "气压" {
            n234 = Index Array(array=w405, index=1 ("索引")) -> (element=w404:string)
          }
          frame "", Default {
            n235 = Index Array(array=w411, index #1=3 ("索引"), index #2=5 ("索引")) -> (element #1=w410:string, element #2=w408:string)
          }
        }
        n236 = Empty String/Path?(string/path=w378) -> (empty?=w379:bool)
        n237 = case shown="False" w379 {
          tunnel: w378 -> [w393 w395]
          tunnel: w376 -> [w392 _]
          tunnel: [w390 w395] -> w377
          frame False {
            n238 = Fract/Exp String To Number(string=w393) -> (number=w394:dbl)  [unwired: 3 in, 1 out]
            n239 = Multiply(x=w394, y=w392) -> (x*y=w391:dbl)
            n240 = Number To Fractional String(number=w391) -> (F-format string=w390:string)  [unwired: 3 in]
          }
          frame True {
            # "空"
          }
        }
        n241 = global read "断电保存全局.vi" "数据发送协议"() -> (w382:enum16{"2005-212协议", "2017-212协议"})
        n242 = call "数据编码整合输出.vi"("table"=w374, "数据标识"=w385, "数据类型"="-Rtd=", "污染物编码"=w373, "地表水/污染源"=FALSE, "数据值"=w377) -> ("编码输出"=w381:string)  [unwired: 5 in]
        n243 = case shown="\"2017-212协议\"" w382 {
          tunnel: w374 -> [w415 _]
          tunnel: w381 -> [w413 w420]
          tunnel: [w414 w420] -> w380
          frame "2005-212协议", Default {
            n244 = case shown="\"假\", Default" w415 {
              tunnel: [w416 "" "" ""] -> w414
              tunnel: w413 -> [w416 _ _ _]
              frame "假", Default {
              }
              frame "分钟雨量", "空气温度", "累积雨量", "日雨量", "相对湿度", "小时雨量" {
              }
              frame "风速", "风向", "气温", "气压" {
              }
              frame "方向", "负累积流量", "累积流量", "流速", "水位", "瞬时流量", "正累积流量" {
              }
            }
          }
          frame "2017-212协议" {
          }
        }
        n245 = Concatenate Strings(w384, w380) -> (w383:string)
      }
      frame "平行样测试" {
        n246 = global read "全局 小时数据发送次数.vi" "小时数据发送次数"() -> (w421:i32)
        n247 = call "平行样集成干预数据组合(子VI).vi"("污染物编码"=w422, "数据输入"=w423, "小时数据发送次数"=w421) -> ("输出组合"=w425:string)  [unwired: 8 in]
        n248 = Concatenate Strings(w426, w425) -> (w424:string)
      }
      frame "集成干预测试" {
        n249 = global read "断电保存全局.vi" "应用环境"() -> (w429:T5)
        n250 = case shown="\"GB212\", Default" w429 {
          tunnel: w433 -> [w437 w443]
          tunnel: w432 -> [w436 w444]
          tunnel: w431 -> [w435 w445]
          tunnel: [w434 w441] -> w430
          tunnel: w428 -> [_ w442]
          tunnel: w427 -> [_ w440]
          frame "STD" {
            n251 = global read "全局 小时数据发送次数.vi" "小时数据发送次数"() -> (w438:i32)
            n252 = call "平行样集成干预数据组合(子VI).vi"("污染物编码"=w437, "数据输入"=w436, "小时数据发送次数"=w438) -> ("输出组合"=w439:string)  [unwired: 8 in]
            n253 = Concatenate Strings(w435, w439) -> (w434:string)
          }
          frame "GB212", Default {
            n254 = global read "全局 小时数据发送次数.vi" "小时数据发送次数"() -> (w456:i32)
            n255 = Index Array(array=w444, index (row)=w456) -> (element=w455:string[])  [unwired: 1 in]
            n256 = case shown="\"\", Default" w440 {
              tunnel: w455 -> [w466 w469]
              tunnel: [w463 w468] -> w448
              tunnel: ["N" ("字符串") w467] -> w453
              frame "风速", "风向", "累积流量", "流速", "气温", "气压", "水位", "瞬时流量" {
                n257 = Index Array(array=w466, index=1 ("索引")) -> (element=w463:string)
              }
              frame "", Default {
                n258 = Index Array(array=w469, index #1=2 ("索引"), index #2=3 ("索引"), index #3=5 ("索引")) -> (element #1=w472:string, element #2=w471:string, element #3=w467:string)
                n259 = case shown="\"N\", Default" w472 {
                  tunnel: [w475 ""] -> w468
                  tunnel: w471 -> [w475 _]
                  frame "N", Default {
                  }
                  frame "M" {
                  }
                }
              }
            }
            n260 = Empty String/Path?(string/path=w448) -> (empty?=w449:bool)
            n261 = case shown="False" w449 {
              tunnel: w448 -> [w460 w462]
              tunnel: w442 -> [w459 _]
              tunnel: [w457 w462] -> w447
              frame False {
                n262 = Fract/Exp String To Number(string=w460) -> (number=w461:dbl)  [unwired: 3 in, 1 out]
                n263 = Multiply(x=w461, y=w459) -> (x*y=w458:dbl)
                n264 = Number To Fractional String(number=w458) -> (F-format string=w457:string)  [unwired: 3 in]
              }
              frame True {
                # "空"
              }
            }
            n265 = global read "断电保存全局.vi" "地表水/污染源"() -> (w446:bool)
            n266 = global read "断电保存全局.vi" "数据发送协议"() -> (w452:enum16{"2005-212协议", "2017-212协议"})
            n267 = call "数据编码整合输出.vi"("table"=w440, "数据标识"=w453, "数据类型"="-Avg=", "污染物编码"=w443, "地表水/污染源"=w446, "数据值"=w447) -> ("编码输出"=w451:string)  [unwired: 5 in]
            n268 = case shown="\"2017-212协议\"" w452 {
              tunnel: w440 -> [w479 _]
              tunnel: w451 -> [w477 w482]
              tunnel: [w478 w482] -> w450
              frame "2005-212协议", Default {
                n269 = case shown="\"假\", Default" w479 {
                  tunnel: [w480 ""] -> w478
                  tunnel: w477 -> [w480 _]
                  frame "假", Default {
                  }
                  frame "风速", "风向", "累积流量", "流速", "气温", "气压", "水位" {
                  }
                }
              }
              frame "2017-212协议" {
              }
            }
            n270 = Concatenate Strings(w445, w450) -> (w441:string)
          }
        }
      }
      frame "加标回收测试" {
        n271 = global read "全局 小时数据发送次数.vi" "小时数据发送次数"() -> (w486:i32)
        n272 = call "加标回收数据组合 (子VI).vi"("小时数据发送次数"=w486, "数据"=w487, "污染物编码"=w483) -> ("组合输出"=w485:string)  [unwired: 7 in, 1 out]
        n273 = Concatenate Strings(w484, w485) -> (w488:string)
      }
      frame "核查数据" {
        n274 = global read "全局 小时数据发送次数.vi" "小时数据发送次数"() -> (w494:i32)
        n275 = call "标样核查数据组合(子VI).vi"("小时数据发送次数"=w494, "数据输入"=w493, "污染物编码"=w492) -> ("输出组合"=w490:string)  [unwired: 8 in]
        n276 = Concatenate Strings(w491, w490) -> (w489:string)
      }
      frame "空白零点跨度数据" {
        n277 = global read "全局 小时数据发送次数.vi" "小时数据发送次数"() -> (w507:i32)
        n278 = Index Array(array=w505, index (row)=w507) -> (element=w511:string[])  [unwired: 1 in]
        n279 = Index Array(array=w511, index #1=0 ("索引"), index #2=3 ("索引"), index #3=6 ("索引"), index #4=7 ("索引"), index #5=5 ("索引")) -> (element #2=w506:string, element #3=w508:string, element #4=w497:string, element #5=w495:string)  [unwired: 1 out]
        n280 = Empty String/Path?(string/path=w497) -> (empty?=w499:bool)
        n281 = case shown="False" w499 {
          tunnel: [w513 "0" ("span value")] -> w498
          tunnel: w497 -> [w513 _]
          frame False {
          }
          frame True {
          }
        }
        n282 = call "零点跨度数据组合 (子VI).vi"("数据标识"=w495, "span value"=w498, "standard value"=w508, "check value"=w506, "污染物编码"=w504) -> ("组合输出"=w503:string)  [unwired: 6 in]
        n283 = Concatenate Strings(w502, w503) -> (w501:string)
      }
      frame "提取小时数据" {
        n284 = global read "全局 小时数据发送次数.vi" "小时数据发送次数"() -> (w531:i32)
        n285 = Index Array(array=w530, index (row)=w531) -> (element=w529:string[])  [unwired: 1 in]
        n286 = Index Array(array=w529, index #2=1 ("索引")) -> (element #2=w518:string)  [unwired: 1 in, 1 out]
        n287 = Empty String/Path?(string/path=w518) -> (empty?=w520:bool)
        n288 = case shown="False" w520 {
          tunnel: w518 -> [w536 w538]
          tunnel: w517 -> [w535 _]
          tunnel: [w533 w538] -> w519
          frame False {
            n289 = Fract/Exp String To Number(string=w536) -> (number=w537:dbl)  [unwired: 3 in, 1 out]
            n290 = Multiply(x=w537, y=w535) -> (x*y=w534:dbl)
            n291 = Number To Fractional String(number=w534) -> (F-format string=w533:string)  [unwired: 3 in]
          }
          frame True {
            # "空"
          }
        }
        n292 = global read "断电保存全局.vi" "地表水/污染源"() -> (w516:bool)
        n293 = global read "断电保存全局.vi" "数据发送协议"() -> (w526:enum16{"2005-212协议", "2017-212协议"})
        n294 = call "数据编码整合输出.vi"("table"=w515, "数据标识"="N", "数据类型"="-Avg=", "污染物编码"=w524, "地表水/污染源"=w516, "数据值"=w519) -> ("编码输出"=w523:string)  [unwired: 5 in]
        n295 = case shown="\"2005-212协议\", Default" w526 {
          tunnel: w524 -> [w541 _]
          tunnel: w523 -> [w539 w544]
          tunnel: [w540 w544] -> w525
          frame "2005-212协议", Default {
            n296 = case shown="\"累积流量\", \"流速\", \"水位\"" w541 {
              tunnel: [w542 ""] -> w540
              tunnel: w539 -> [w542 _]
              frame "假", Default {
              }
              frame "累积流量", "流速", "水位" {
              }
            }
          }
          frame "2017-212协议" {
          }
        }
        n297 = Concatenate Strings(w522, w525) -> (w521:string)
      }
      frame "提取实时数据" {
        n298 = global read "全局 小时数据发送次数.vi" "小时数据发送次数"() -> (w560:i32)
        n299 = Index Array(array=w553, index (row)=w560) -> (element=w561:string[])  [unwired: 1 in]
        n300 = Index Array(array=w561, index #1=3 ("索引"), index #2=5 ("索引")) -> (element #1=w548:string, element #2=w558:string)
        n301 = Empty String/Path?(string/path=w548) -> (empty?=w550:bool)
        n302 = case shown="False" w550 {
          tunnel: w548 -> [w567 w569]
          tunnel: w547 -> [w566 _]
          tunnel: [w564 w569] -> w549
          frame False {
            n303 = Fract/Exp String To Number(string=w567) -> (number=w568:dbl)  [unwired: 3 in, 1 out]
            n304 = Multiply(x=w568, y=w566) -> (x*y=w565:dbl)
            n305 = Number To Fractional String(number=w565) -> (F-format string=w564:string)  [unwired: 3 in]
          }
          frame True {
            # "空"
          }
        }
        n306 = global read "断电保存全局.vi" "地表水/污染源"() -> (w546:bool)
        n307 = global read "断电保存全局.vi" "数据发送协议"() -> (w557:enum16{"2005-212协议", "2017-212协议"})
        n308 = call "数据编码整合输出.vi"("table"=w545, "数据标识"=w558, "数据类型"="-Rtd=", "污染物编码"=w552, "地表水/污染源"=w546, "数据值"=w549) -> ("编码输出"=w556:string)  [unwired: 5 in]
        n309 = case shown="\"2017-212协议\"" w557 {
          tunnel: w552 -> [w572 _]
          tunnel: w556 -> [w570 w575]
          tunnel: [w571 w575] -> w555
          frame "2005-212协议", Default {
            n310 = case shown="\"累积流量\", \"流速\", \"水位\"" w572 {
              tunnel: [w573 ""] -> w571
              tunnel: w570 -> [w573 _]
              frame "假", Default {
              }
              frame "累积流量", "流速", "水位" {
              }
            }
          }
          frame "2017-212协议" {
          }
        }
        n311 = Concatenate Strings(w554, w555) -> (w551:string)
      }
      frame "操作日志" {
        n312 = global read "断电保存全局.vi" "因子编码簇"() -> (w581:T4)
        n313 = global read "全局 小时数据发送次数.vi" "小时数据发送次数"() -> (w594:i32)
        n314 = Unbundle By Name(w581) -> ("DO"=w580:string)
        n315 = Equal?(x=w578, y=w580) -> (x = y?=w576:bool)
        n316 = Index Array(array=w590, index (row)=w594) -> (element=w589:string[])  [unwired: 1 in]
        n317 = Index Array(array=w589, index #1=0 ("索引"), index #2=2 ("索引")) -> (element #2=w588:string)  [unwired: 1 out]
        n318 = Empty String/Path?(string/path=w588) -> (empty?=w593:bool)
        n319 = Select(t="w00000", s=w576, f=w578) -> (s? t:f=w577:string)
        n320 = Select(t="i21001", s=w576, f="i11001") -> (s? t:f=w582:string)
        n321 = case shown="False" w593 {
          tunnel: [w598 ""] -> w587
          tunnel: w588 -> [w596 _]
          tunnel: w577 -> [w597 _]
          tunnel: w582 -> [w595 _]
          frame False {
            n322 = Format Into String(format string="PolId=%s,%s-Info=//%s//;" ("格式字符串"), w597, w595, w596) -> (resulting string=w598:string)  [unwired: 2 in, 1 out]
          }
          frame True {
          }
        }
        n323 = Concatenate Strings(w586, w587) -> (w585:string)
      }
      frame "仪器参数" {
        n324 = global read "断电保存全局.vi" "应用环境"() -> (w602:T5)
        n325 = global read "全局 小时数据发送次数.vi" "小时数据发送次数"() -> (w609:i32)
        n326 = case shown="\"GB212\", Default" w602 {
          tunnel: ["3090仪器参数" ("table") "仪器参数" ("table")] -> w601
          frame "STD" {
          }
          frame "GB212", Default {
          }
        }
        n327 = Index Array(array=w608, index (row)=w609) -> (element=w607:string[])  [unwired: 1 in]
        n328 = call "关键参数组合 (子VI).vi"("table"=w601, "因子编码"=w606, "data"=w607) -> ("字符串"=w605:string)  [unwired: 8 in]
        n329 = Concatenate Strings(w604, w605) -> (w603:string)
      }
      frame "3090仪器参数" {
        n330 = global read "全局 小时数据发送次数.vi" "小时数据发送次数"() -> (w619:i32)
        n331 = Index Array(array=w615, index (row)=w619) -> (element=w617:string[])  [unwired: 1 in]
        n332 = call "关键参数组合 (子VI).vi"("table"="3090仪器参数", "因子编码"=w613, "data"=w617) -> ("字符串"=w616:string)  [unwired: 8 in]
        n333 = Concatenate Strings(w614, w616) -> (w612:string)
      }
      frame "提取仪器参数" {
        n334 = global read "全局 小时数据发送次数.vi" "小时数据发送次数"() -> (w626:i32)
        n335 = Index Array(array=w625, index (row)=w626) -> (element=w623:string[])  [unwired: 1 in]
        n336 = call "提取仪器参数 (子VI).vi"("因子编码"=w624, "数据输入"=w623) -> ("字符串"=w622:string)  [unwired: 9 in]
        n337 = Concatenate Strings(w621, w622) -> (w620:string)
      }
      frame "报警信息" {
        n338 = Empty String/Path?(string/path=w631) -> (empty?=w630:bool)
        n339 = global read "断电保存全局.vi" "因子编码簇"() -> (w653:T4)
        n340 = case shown="\"CODMn\"" w645 {
          tunnel: [u16 0 ("register") w671 w677 w683 w689 w695] -> w643
          tunnel: [u16 0 ("register") w668 w674 w680 w686 w692] -> w628
          frame "假", Default {
          }
          frame "CODMn" {
            n341 = global read "全局1.vi" "读取试剂余量的值"() -> (w669:u16[])
            n342 = global read "全局1.vi" "register values"() -> (w673:u16[])
            n343 = Index Array(array=w673, index=1 ("索引")) -> (element=w671:u16)
            n344 = Index Array(array=w669, index=0 ("索引")) -> (element=w668:u16)
          }
          frame "氨氮" {
            n345 = global read "全局1.vi" "读取试剂余量的值"() -> (w675:u16[])
            n346 = global read "全局1.vi" "register values"() -> (w679:u16[])
            n347 = Index Array(array=w679, index=2 ("索引")) -> (element=w677:u16)
            n348 = Index Array(array=w675, index=1 ("索引")) -> (element=w674:u16)
          }
          frame "总磷" {
            n349 = global read "全局1.vi" "读取试剂余量的值"() -> (w681:u16[])
            n350 = global read "全局1.vi" "register values"() -> (w685:u16[])
            n351 = Index Array(array=w685, index=3 ("索引")) -> (element=w683:u16)
            n352 = Index Array(array=w681, index=2 ("索引")) -> (element=w680:u16)
          }
          frame "总氮" {
            n353 = global read "全局1.vi" "读取试剂余量的值"() -> (w687:u16[])
            n354 = global read "全局1.vi" "register values"() -> (w691:u16[])
            n355 = Index Array(array=w691, index=4 ("索引")) -> (element=w689:u16)
            n356 = Index Array(array=w687, index=3 ("索引")) -> (element=w686:u16)
          }
          frame "CODCr" {
            n357 = global read "全局1.vi" "读取试剂余量的值"() -> (w693:u16[])
            n358 = global read "全局1.vi" "register values"() -> (w697:u16[])
            n359 = Index Array(array=w697, index=5 ("索引")) -> (element=w695:u16)
            n360 = Index Array(array=w693, index=4 ("索引")) -> (element=w692:u16)
          }
        }
        n361 = global read "全局 小时数据发送次数.vi" "小时数据发送次数"() -> (w648:i32)
        n362 = Unbundle By Name(w653) -> ("藻密度"=w652:string)
        n363 = Equal?(x=w650, y=w652) -> (x = y?=w640:bool)
        n364 = Index Array(array=w647, index (row)=w648) -> (element=w646:string[])  [unwired: 1 in]
        n365 = Select(t="w00000", s=w640, f=w650) -> (s? t:f=w649:string)
        n366 = Index Array(array=w646, index #1=0 ("索引"), index #2=2 ("索引")) -> (element #1=w627:string, element #2=w659:string)
        n367 = Empty String/Path?(string/path=w627) -> (empty?=w658:bool)
        n368 = Select(t="i22001", s=w640, f="i12001") -> (s? t:f=w639:string)
        n369 = Select(t="i22003", s=w640, f="i12031") -> (s? t:f=w638:string)
        n370 = Number To Decimal String(number=w643) -> (decimal integer string=w644:string)  [unwired: 1 in]
        n371 = Number To Decimal String(number=w628) -> (decimal integer string=w629:string)  [unwired: 1 in]
        n372 = case shown="False" w658 {
          tunnel: [w706 _] -> w635
          tunnel: w659 -> [w703 _]
          tunnel: w649 -> [w701 _]
          tunnel: w644 -> [w699 _]
          tunnel: w639 -> [w700 _]
          tunnel: w638 -> [w704 _]
          tunnel: w629 -> [w698 _]
          frame False {
            n373 = call "告警信息文本转换为协议i12031值.vi"("字符串"=w703) -> ("十进制整型字符串"=w702:string)  [unwired: 10 in]
            n374 = Format Into String(format string="PolId=%s,%s-Info=%s,i12002-Info=0,i12003-Info=%s,%s-Info=%s;" ("格式字符串"), w701, w700, w699, w698, w704, w702) -> (resulting string=w706:string)  [unwired: 2 in, 1 out]
          }
          frame True {
          }
        }
        n375 = Empty String/Path?(string/path=w635) -> (empty?=w634:bool)
        n376 = Concatenate Strings(w631, w635) -> (w637:string)
        n377 = Not(x=w634) -> (.not. x?=w633:bool)
        n378 = And(x=w630, y=w633) -> (x .and. y?=w632:bool)
        n379 = case shown="True" w632 {
          tunnel: w627 -> [_ w663]
          tunnel: w637 -> [w660 w662]
          tunnel: [w660 w661] -> w636
          frame False {
          }
          frame True {
            n380 = call "规范时间戳.vi"("字符串"=w663) -> ("result string"=w665:string)  [unwired: 10 in]
            n381 = Format Into String(format string="DataTime=%s;%s", w665, w662) -> (resulting string=w661:string)  [unwired: 2 in, 1 out]
          }
        }
      }
    }
  }
  "字符串" <- w46
